vi "Assignment.vi"() -> ()   [LabVIEW 2023]
uses:
  Control 1.ctl
  Control 2.ctl
panel:
  in  "Tab Control":enum32{"Page 1", "Page 2", "Page 3"}(tab)
  out "seconds":string
  out "welcome":string
  out "Move Back":bool
  out "Move Forward":bool
  out "Vehicle Out of Position":bool
  out "Air Dry":bool
  out "Clear Water Rinse":bool
  out "Main High Pressure Wash":bool
  out "Soap Application":bool
  out "Under Body Wash":bool
  in  "Air Dry\nPosition \nSwitch":bool
  in  "Main Wash\nPosition\nSwitch":bool
  in  "Under Body\nWash Position\nSwitch":bool
  in  "Economy Wash":bool
  in  "Deluxe Wash":bool
  in  "stop":bool
  out "Next cycle in:":dbl format="%#.2f"
  out "Current Cycle:":string
  in  "Guest":bool
  in  "Login":bool
  in  "Password:":string
  in  "Username:":string
  # "Car Wash indicators"
  # "Car Wash Simulation Switches"
  # "Purchase Selection"
  # "Welcome to Touchless Carwash"
  # "Wash Complete! Drive Safely."
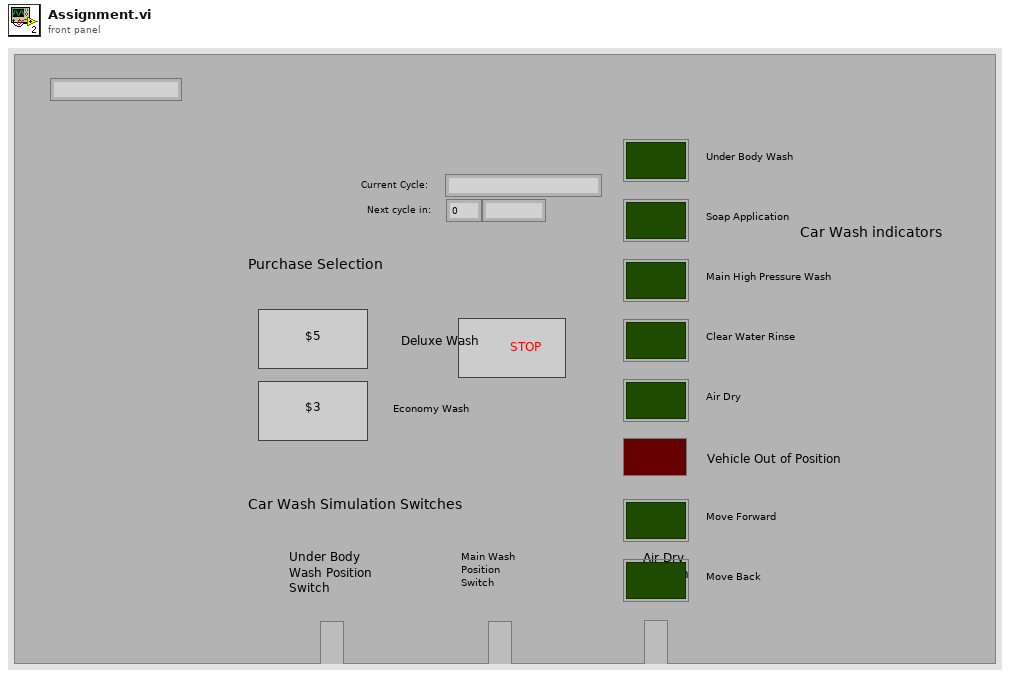
[diagram p1: front panel]
types:
  T1 = typedef "Control 1.ctl" = enum16{"init", "Login", "monitor switch", "monitor purchase selection", "decrement timer cycle", "Update cycle", "Logging"}
  T2 = enum8{"Enabled", "Disabled", "Disabled and Grayed Out"}
  T3 = typedef "Control 2.ctl" = enum16{"Under Body Wash", "Soap Application", "Main High Pressure Wash", "Clear Water Rinse", "Air Dry"}
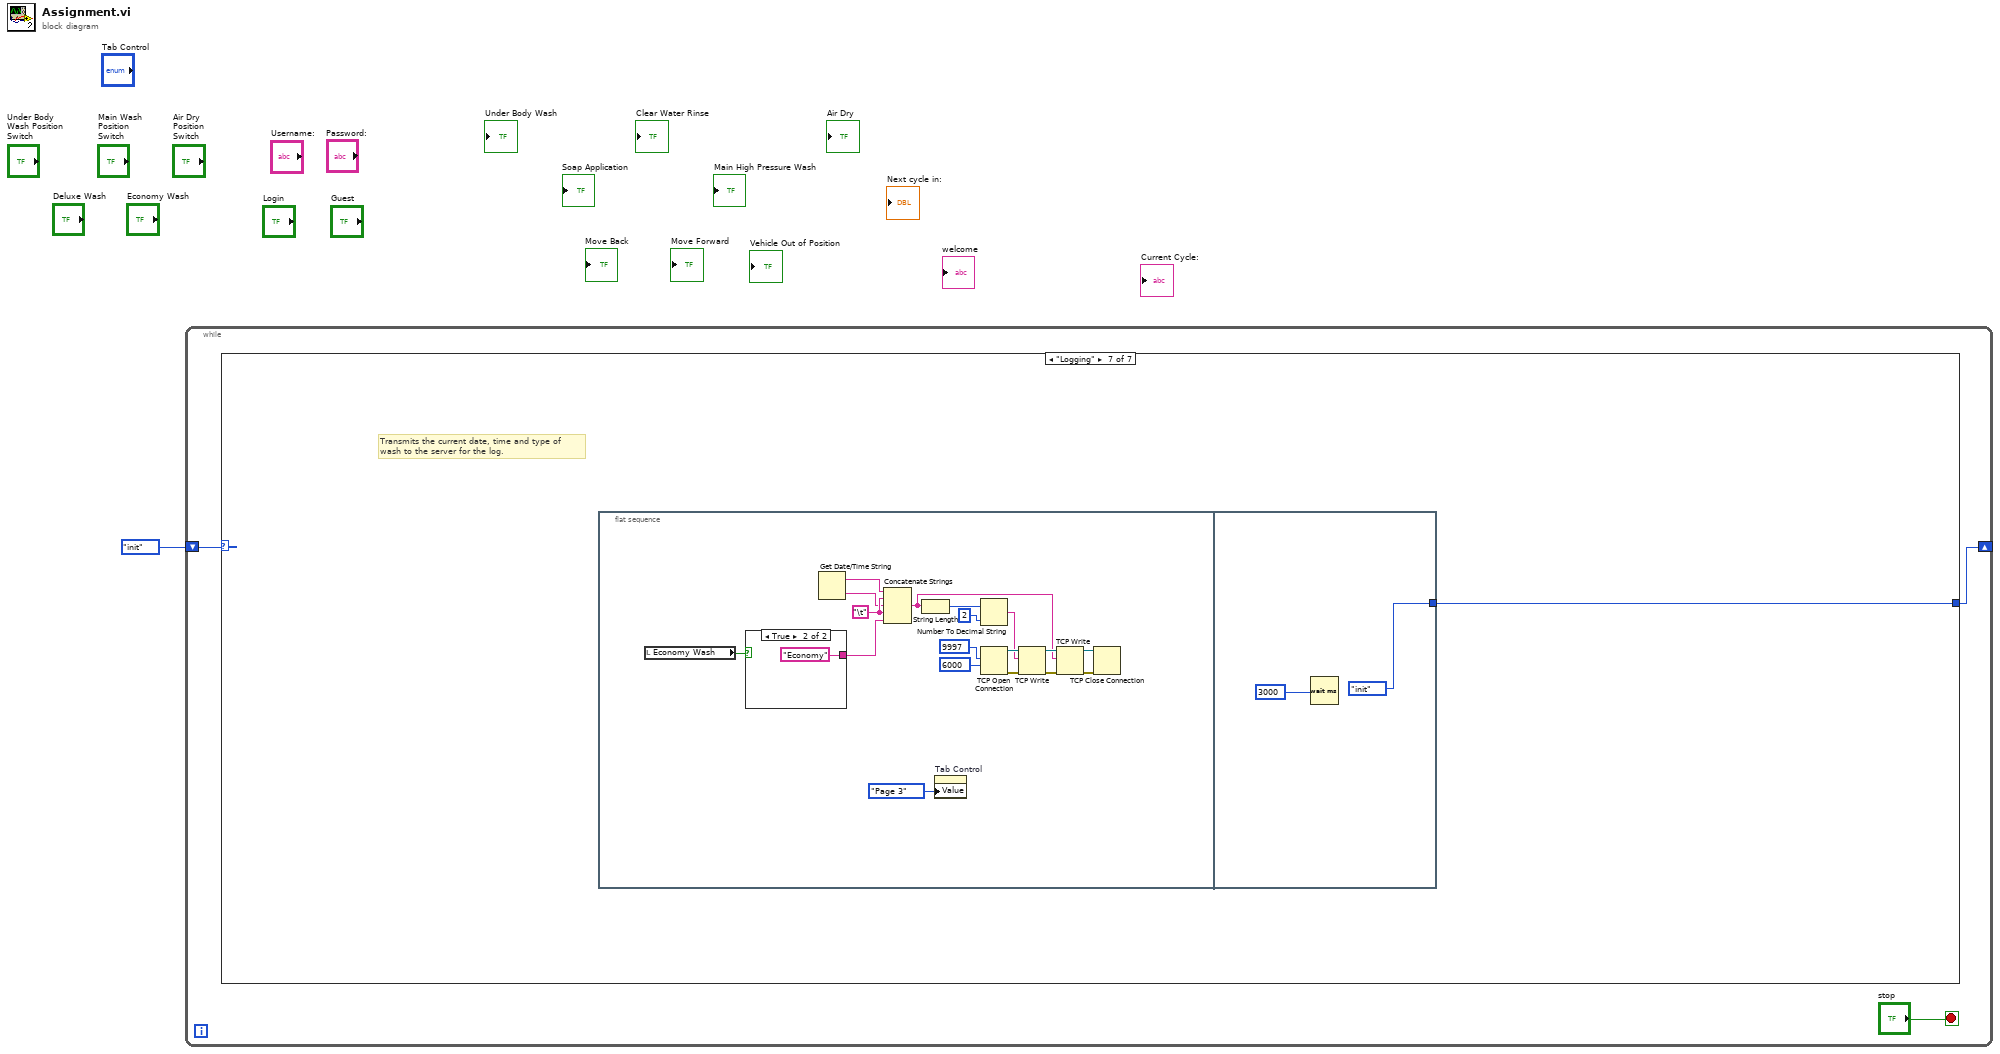
[diagram p0: block diagram]
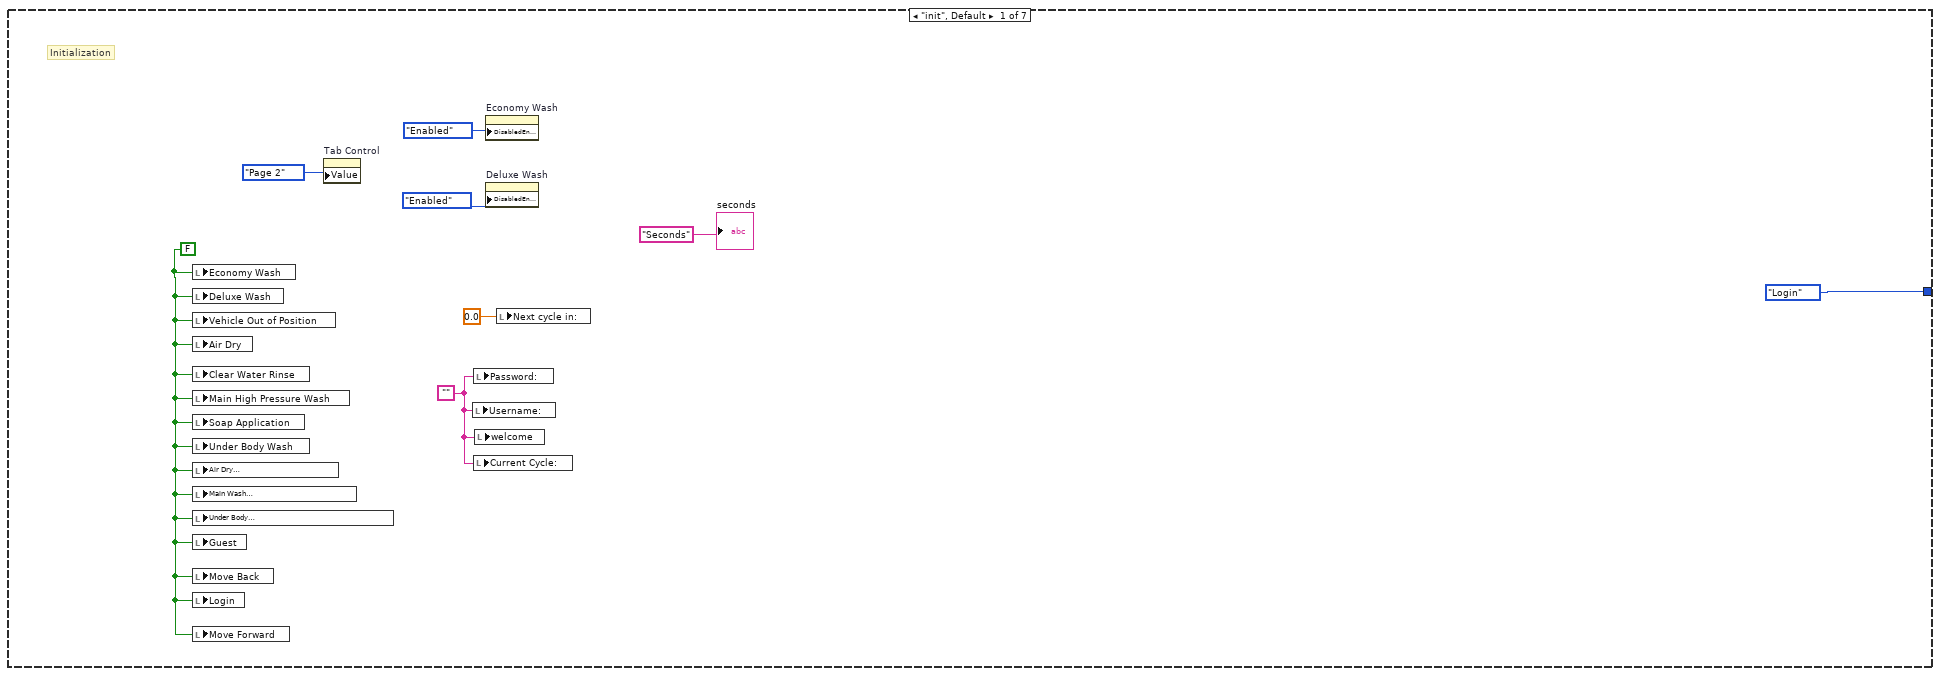
[diagram p2: hidden frame]
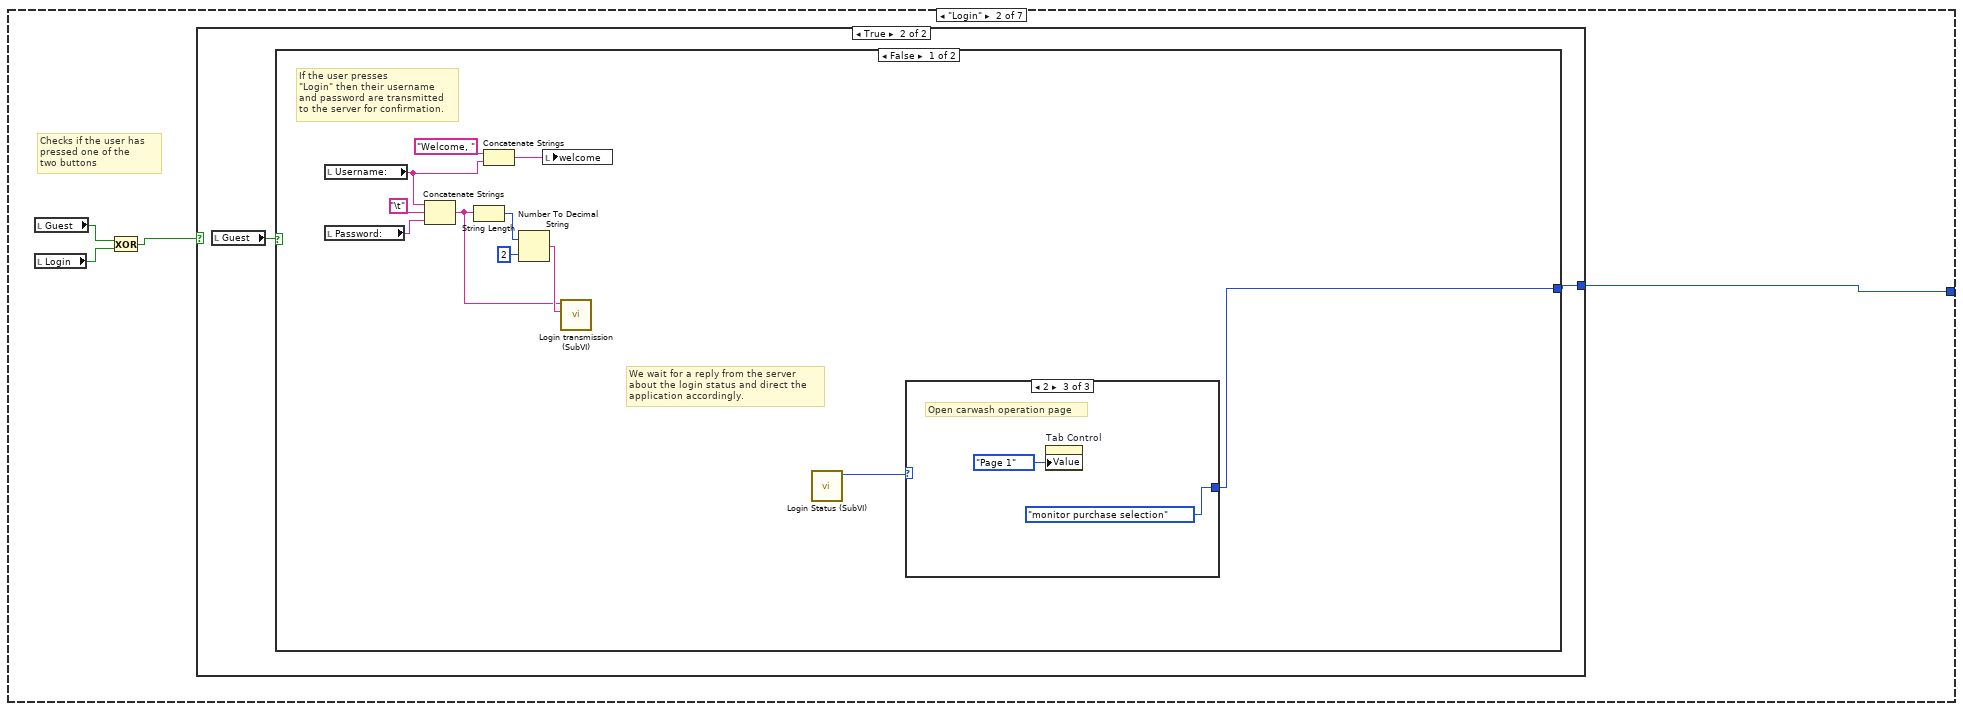
[diagram p3: hidden frame]
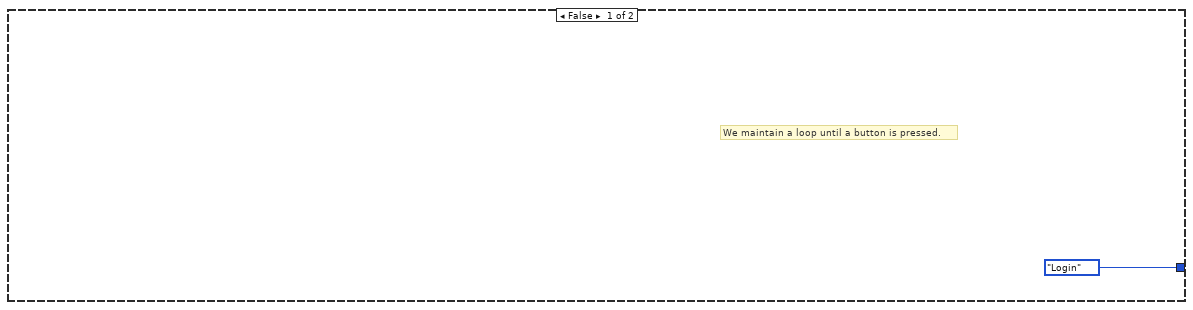
[diagram p4: hidden frame]
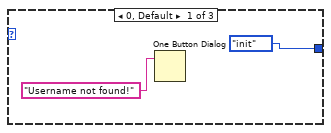
[diagram p5: hidden frame]
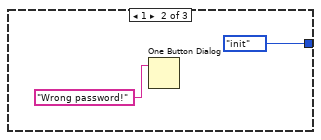
[diagram p6: hidden frame]
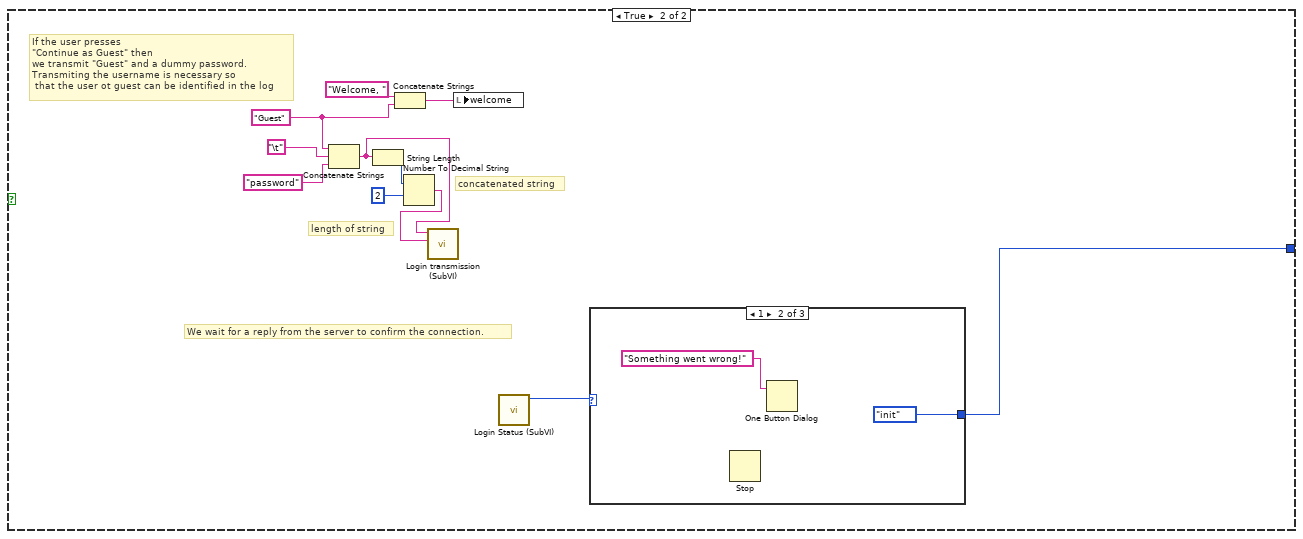
[diagram p7: hidden frame]
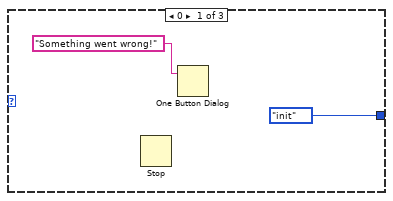
[diagram p8: hidden frame]
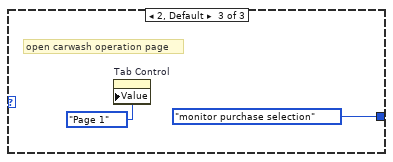
[diagram p9: hidden frame]
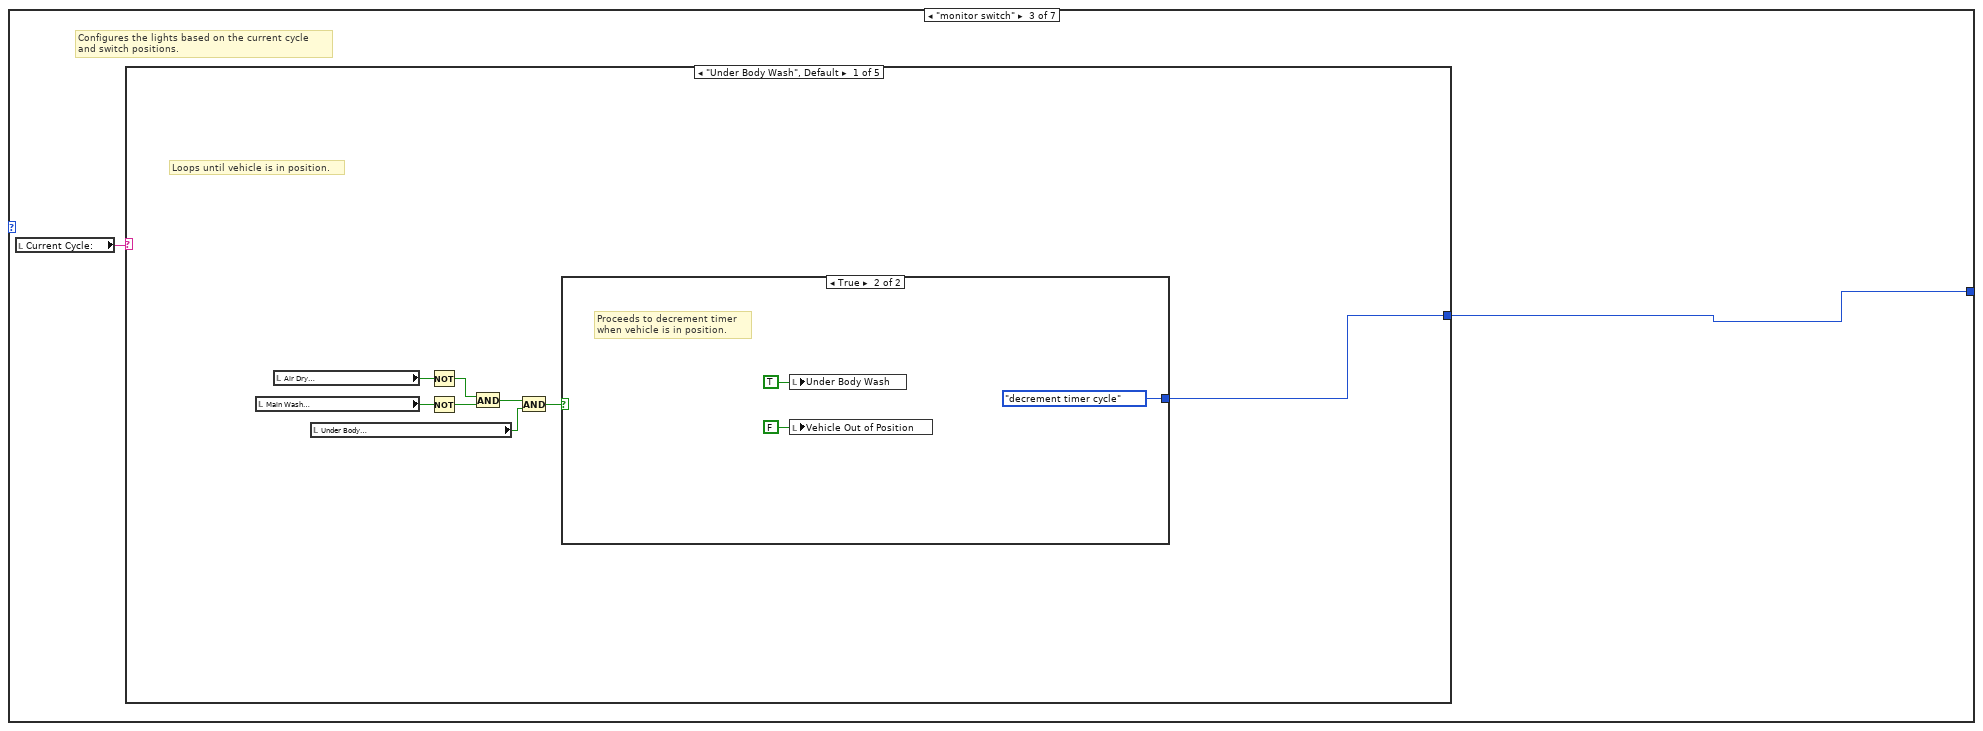
[diagram p10: hidden frame]
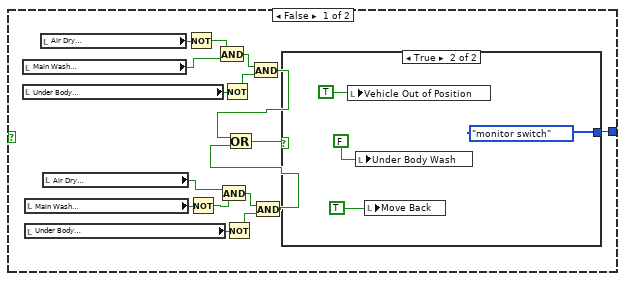
[diagram p11: hidden frame]
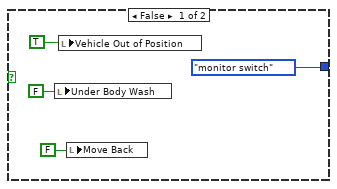
[diagram p12: hidden frame]
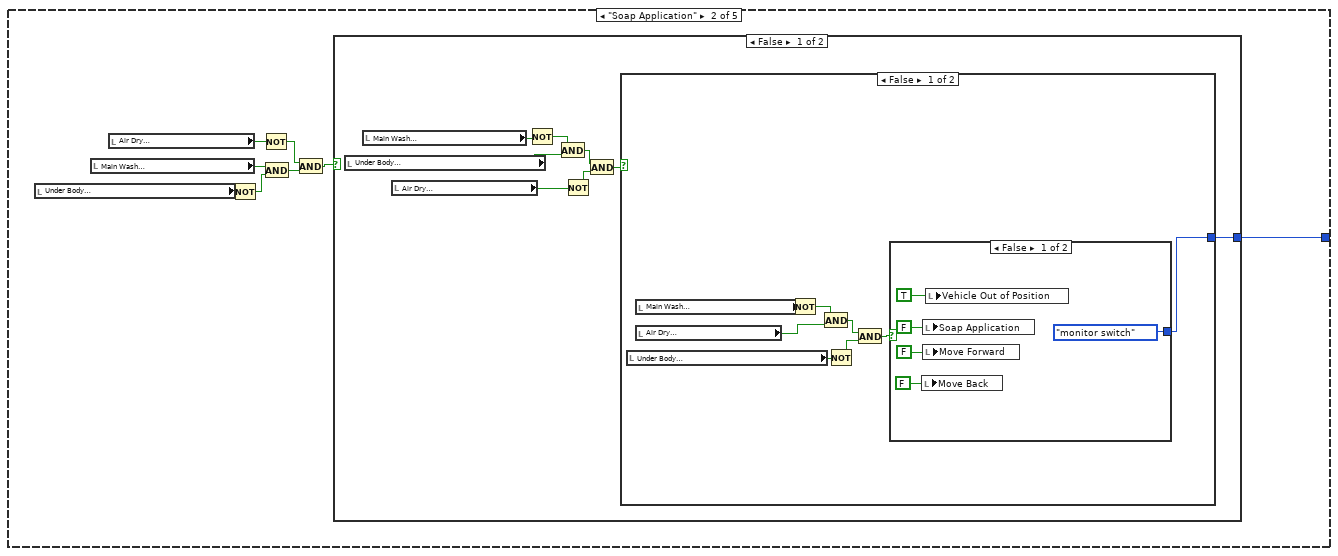
[diagram p13: hidden frame]
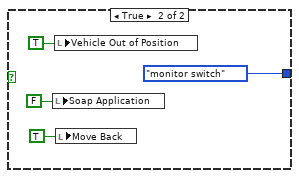
[diagram p14: hidden frame]
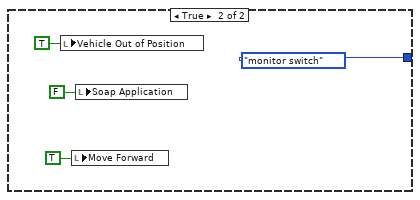
[diagram p15: hidden frame]
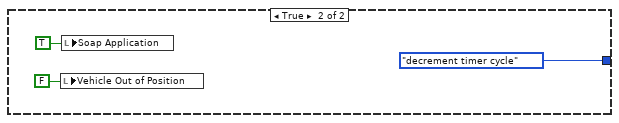
[diagram p16: hidden frame]
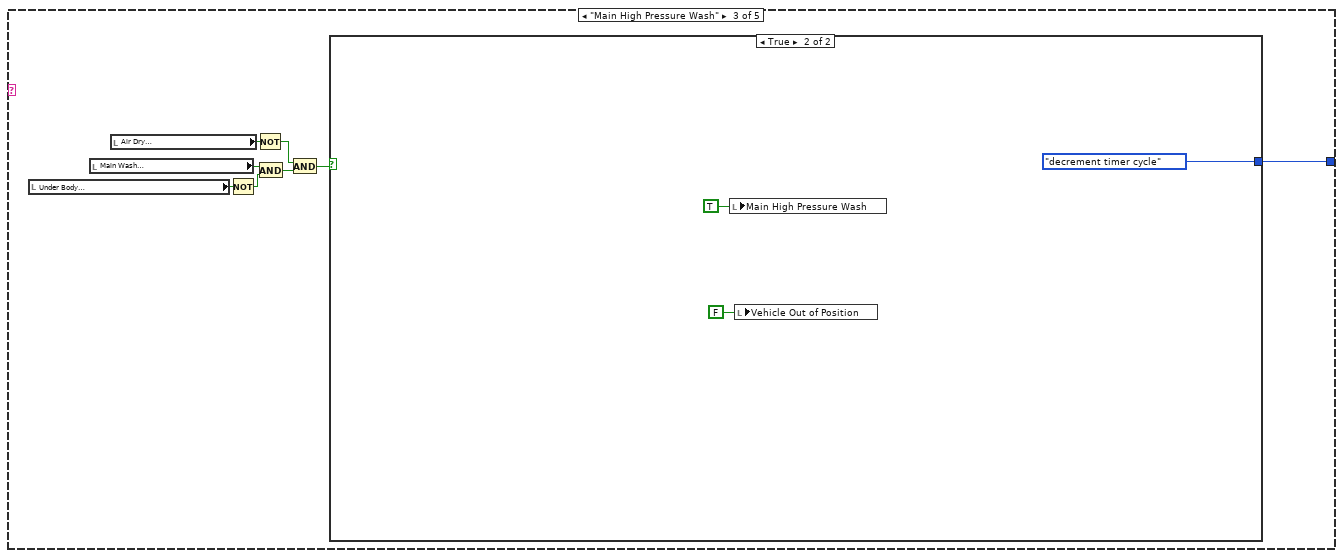
[diagram p17: hidden frame]
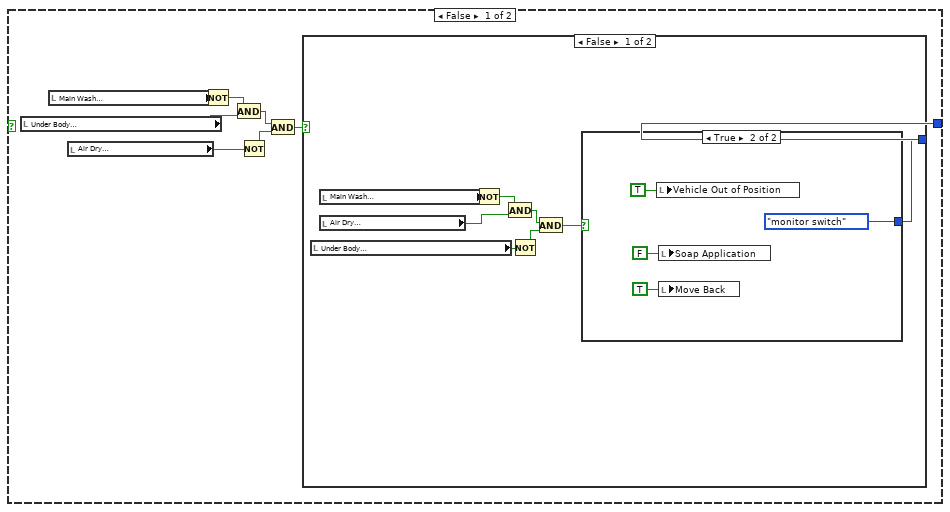
[diagram p18: hidden frame]
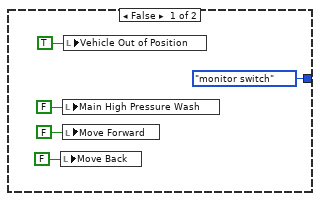
[diagram p19: hidden frame]
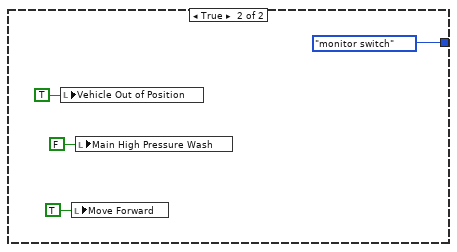
[diagram p20: hidden frame]
diagram:
  n1 = while {
    shift-right: [w3] -> _
    shift-left: Control_1."init" -> [w2]
    stop <- "stop" stop-if-true
    n2 = case shown="\"Logging\"" w2 {
      tunnel: [Control_1."Login" w13 w55 w246 Control_1."Update cycle" w270 w301] -> w3
      frame "init", Default {
        w5 = ""
        w7 = FALSE
        # "Initialization"
        n3 = local write "Economy Wash"(w7) -> ()
        n4 = local write "Deluxe Wash"(w7) -> ()
        n5 = local write "Vehicle Out of Position"(w7) -> ()
        n6 = local write "Air Dry"(w7) -> ()
        n7 = local write "Clear Water Rinse"(w7) -> ()
        n8 = local write "Main High Pressure Wash"(w7) -> ()
        n9 = local write "Soap Application"(w7) -> ()
        n10 = local write "Under Body Wash"(w7) -> ()
        n11 = local write "Air Dry\nPosition \nSwitch"(w7) -> ()
        n12 = local write "Main Wash\nPosition\nSwitch"(w7) -> ()
        n13 = local write "Under Body\nWash Position\nSwitch"(w7) -> ()
        n14 = local write "Guest"(w7) -> ()
        n15 = local write "Move Back"(w7) -> ()
        n16 = local write "Login"(w7) -> ()
        n17 = local write "Move Forward"(w7) -> ()
        n18 = property on="Tab Control" class="TabCtl (strict)"("Value"=enum32{"Page 1", "Page 2"}."Page 2" ("Tab Control")) -> ()  [unwired: 2 in, 2 out]
        n19 = local write "Username:"(w5) -> ()
        n20 = local write "Password:"(w5) -> ()
        n21 = local write "Current Cycle:"(w5) -> ()
        n22 = local write "welcome"(w5) -> ()
        n23 = property on="Economy Wash" class="Bool (strict)"("DisabledEnum"=T2."Enabled" ("Disabled")) -> ()  [unwired: 2 in, 2 out]
        n24 = property on="Deluxe Wash" class="Bool (strict)"("DisabledEnum"=T2."Enabled" ("Disabled")) -> ()  [unwired: 2 in, 2 out]
        n25 = local write "Next cycle in:"(0.0 ("Timer")) -> ()
        "seconds" <- "Seconds" ("seconds")
      }
      frame "Login" {
        # "Checks if the user has \npressed one of the\ntwo buttons"
        n26 = local read "Guest"() -> (w15:bool)
        n27 = local read "Login"() -> (w14:bool)
        n28 = Exclusive Or(1:w14, 2:w15) -> (0:w16:bool)
        n29 = case shown="True" w16 {
          tunnel: [Control_1."Login" w18] -> w13
          frame False {
            # "We maintain a loop until a button is pressed."
          }
          frame True {
            n30 = local read "Guest"() -> (w19:bool)
            n31 = case shown="False" w19 {
              tunnel: [w26 w43] -> w18
              frame False {
                # "We wait for a reply from the server\nabout the login status and direct the \napplication accordingly."
                # "If the user presses \n\"Login\" then their username \nand password are transmitted\nto the server for confirmation."
                n32 = local read "Username:"() -> (w21:string)
                n33 = local read "Password:"() -> (w30:string)
                n34 = Concatenate Strings(w21, "\t", w30) -> (w24:string)
                n35 = String Length(string=w24) -> (length=w29:i32)
                n36 = Concatenate Strings("Welcome, " ("string"), w21) -> (w22:string)
                n37 = Number To Decimal String(number=w29, width (-)=i16 2) -> (decimal integer string=w28:string)
                n38 = local write "welcome"(w22) -> ()
                n39 = call "Login transmission (SubVI).vi"("length of string"=w28, "String"=w24) -> ()  [unwired: 10 in]
                n40 = call "Login Status (SubVI).vi"() -> ("Numeric"=w20:i32)  [unwired: 11 in]
                n41 = case shown="2" w20 {
                  tunnel: [Control_1."init" Control_1."init" Control_1."monitor purchase selection"] -> w26
                  frame 0, Default {
                    n42 = One Button Dialog(message="Username not found!") -> ()  [unwired: 1 in, 1 out]
                  }
                  frame 1 {
                    n43 = One Button Dialog(message="Wrong password!") -> ()  [unwired: 1 in, 1 out]
                  }
                  frame 2 {
                    # "Open carwash operation page"
                    n44 = property on="Tab Control" class="TabCtl (strict)"("Value"=enum32{"Page 1", "Page 2"}."Page 1" ("Tab Control")) -> ()  [unwired: 2 in, 2 out]
                  }
                }
              }
              frame True {
                w37 = "Guest" ("string")
                # "concatenated string"
                # "length of string"
                # "We wait for a reply from the server to confirm the connection."
                # "If the user presses \n\"Continue as Guest\" then\nwe transmit \"Guest\" and a dummy password.\nTransmiting the username is necessary so\n that the user ot guest can be identified in the log"
                n45 = Concatenate Strings(w37, "\t", "password" ("string")) -> (w40:string)
                n46 = String Length(string=w40) -> (length=w47:i32)
                n47 = Concatenate Strings("Welcome, " ("string"), w37) -> (w39:string)
                n48 = Number To Decimal String(number=w47, width (-)=i16 2) -> (decimal integer string=w41:string)
                n49 = call "Login transmission (SubVI).vi"("length of string"=w41, "String"=w40) -> ()  [unwired: 10 in]
                n50 = local write "welcome"(w39) -> ()
                n51 = call "Login Status (SubVI).vi"() -> ("Numeric"=w46:i32)  [unwired: 11 in]
                n52 = case shown="1" w46 {
                  tunnel: [Control_1."init" Control_1."init" Control_1."monitor purchase selection"] -> w43
                  frame 0 {
                    n53 = Stop() -> ()  [unwired: 1 in]
                    n54 = One Button Dialog(message="Something went wrong!") -> ()  [unwired: 1 in, 1 out]
                  }
                  frame 1 {
                    n55 = Stop() -> ()  [unwired: 1 in]
                    n56 = One Button Dialog(message="Something went wrong!") -> ()  [unwired: 1 in, 1 out]
                  }
                  frame 2, Default {
                    # "open carwash operation page"
                    n57 = property on="Tab Control" class="TabCtl (strict)"("Value"=enum32{"Page 1", "Page 2"}."Page 1" ("Tab Control")) -> ()  [unwired: 2 in, 2 out]
                  }
                }
              }
            }
          }
        }
      }
      frame "monitor switch" {
        # "Configures the lights based on the current cycle\nand switch positions."
        n58 = local read "Current Cycle:"() -> (w54:string)
        n59 = case shown="\"Under Body Wash\", Default" w54 {
          tunnel: [w56 w92 w132 w172 w211] -> w55
          frame "Under Body Wash", Default {
            # "Loops until vehicle is in position."
            n60 = local read "Main Wash\nPosition\nSwitch"() -> (w63:bool)
            n61 = local read "Air Dry\nPosition \nSwitch"() -> (w62:bool)
            n62 = local read "Under Body\nWash Position\nSwitch"() -> (w59:bool)
            n63 = Not(x=w62) -> (.not. x?=w61:bool)
            n64 = Not(x=w63) -> (.not. x?=w60:bool)
            n65 = And(x=w61, y=w60) -> (x .and. y?=w58:bool)
            n66 = And(x=w58, y=w59) -> (x .and. y?=w57:bool)
            n67 = case shown="True" w57 {
              tunnel: [w65 Control_1."decrement timer cycle"] -> w56
              frame False {
                n68 = local read "Main Wash\nPosition\nSwitch"() -> (w76:bool)
                n69 = local read "Under Body\nWash Position\nSwitch"() -> (w79:bool)
                n70 = local read "Main Wash\nPosition\nSwitch"() -> (w70:bool)
                n71 = local read "Under Body\nWash Position\nSwitch"() -> (w71:bool)
                n72 = local read "Air Dry\nPosition \nSwitch"() -> (w78:bool)
                n73 = local read "Air Dry\nPosition \nSwitch"() -> (w69:bool)
                n74 = Not(x=w78) -> (.not. x?=w77:bool)
                n75 = Not(x=w70) -> (.not. x?=w68:bool)
                n76 = And(x=w77, y=w76) -> (x .and. y?=w74:bool)
                n77 = And(x=w69, y=w68) -> (x .and. y?=w73:bool)
                n78 = Not(x=w79) -> (.not. x?=w75:bool)
                n79 = Not(x=w71) -> (.not. x?=w72:bool)
                n80 = And(x=w74, y=w75) -> (x .and. y?=w67:bool)
                n81 = And(x=w73, y=w72) -> (x .and. y?=w66:bool)
                n82 = Or(x=w67, y=w66) -> (x .or. y?=w64:bool)
                n83 = case shown="True" w64 {
                  tunnel: [Control_1."monitor switch" Control_1."monitor switch"] -> w65
                  frame False {
                    n84 = local write "Under Body Wash"(FALSE ("Under Body Wash")) -> ()
                    n85 = local write "Vehicle Out of Position"(TRUE ("Vehicle Out of Position")) -> ()
                    n86 = local write "Move Back"(FALSE ("Move Back")) -> ()
                  }
                  frame True {
                    n87 = local write "Vehicle Out of Position"(TRUE ("Vehicle Out of Position")) -> ()
                    n88 = local write "Under Body Wash"(FALSE ("Under Body Wash")) -> ()
                    n89 = local write "Move Back"(TRUE ("Move Back")) -> ()
                  }
                }
              }
              frame True {
                # "Proceeds to decrement timer\nwhen vehicle is in position."
                n90 = local write "Under Body Wash"(TRUE ("Under Body Wash")) -> ()
                n91 = local write "Vehicle Out of Position"(FALSE ("Vehicle Out of Position")) -> ()
              }
            }
          }
          frame "Soap Application" {
            n92 = local read "Under Body\nWash Position\nSwitch"() -> (w98:bool)
            n93 = local read "Main Wash\nPosition\nSwitch"() -> (w95:bool)
            n94 = local read "Air Dry\nPosition \nSwitch"() -> (w97:bool)
            n95 = Not(x=w98) -> (.not. x?=w96:bool)
            n96 = Not(x=w97) -> (.not. x?=w93:bool)
            n97 = And(x=w95, y=w96) -> (x .and. y?=w94:bool)
            n98 = And(x=w93, y=w94) -> (x .and. y?=w91:bool)
            n99 = case shown="False" w91 {
              tunnel: [w99 Control_1."decrement timer cycle"] -> w92
              frame False {
                n100 = local read "Under Body\nWash Position\nSwitch"() -> (w103:bool)
                n101 = local read "Main Wash\nPosition\nSwitch"() -> (w105:bool)
                n102 = local read "Air Dry\nPosition \nSwitch"() -> (w106:bool)
                n103 = Not(x=w105) -> (.not. x?=w104:bool)
                n104 = And(x=w104, y=w103) -> (x .and. y?=w101:bool)
                n105 = Not(x=w106) -> (.not. x?=w102:bool)
                n106 = And(x=w101, y=w102) -> (x .and. y?=w100:bool)
                n107 = case shown="False" w100 {
                  tunnel: [w108 Control_1."monitor switch"] -> w99
                  frame False {
                    n108 = local read "Under Body\nWash Position\nSwitch"() -> (w109:bool)
                    n109 = local read "Main Wash\nPosition\nSwitch"() -> (w110:bool)
                    n110 = local read "Air Dry\nPosition \nSwitch"() -> (w112:bool)
                    n111 = Not(x=w110) -> (.not. x?=w111:bool)
                    n112 = And(x=w111, y=w112) -> (x .and. y?=w114:bool)
                    n113 = Not(x=w109) -> (.not. x?=w113:bool)
                    n114 = And(x=w114, y=w113) -> (x .and. y?=w107:bool)
                    n115 = case shown="False" w107 {
                      tunnel: [Control_1."monitor switch" Control_1."monitor switch"] -> w108
                      frame False {
                        n116 = local write "Move Back"(FALSE ("Move Back")) -> ()
                        n117 = local write "Soap Application"(FALSE ("Under Body Wash")) -> ()
                        n118 = local write "Move Forward"(FALSE ("Move Back")) -> ()
                        n119 = local write "Vehicle Out of Position"(TRUE ("Vehicle Out of Position")) -> ()
                      }
                      frame True {
                        n120 = local write "Soap Application"(FALSE ("Under Body Wash")) -> ()
                        n121 = local write "Vehicle Out of Position"(TRUE ("Vehicle Out of Position")) -> ()
                        n122 = local write "Move Back"(TRUE ("Move Back")) -> ()
                      }
                    }
                  }
                  frame True {
                    n123 = local write "Vehicle Out of Position"(TRUE ("Vehicle Out of Position")) -> ()
                    n124 = local write "Move Forward"(TRUE ("Move Back")) -> ()
                    n125 = local write "Soap Application"(FALSE ("Under Body Wash")) -> ()
                  }
                }
              }
              frame True {
                n126 = local write "Vehicle Out of Position"(FALSE ("Vehicle Out of Position")) -> ()
                n127 = local write "Soap Application"(TRUE ("Soap Application")) -> ()
              }
            }
          }
          frame "Main High Pressure Wash" {
            n128 = local read "Under Body\nWash Position\nSwitch"() -> (w138:bool)
            n129 = local read "Main Wash\nPosition\nSwitch"() -> (w135:bool)
            n130 = local read "Air Dry\nPosition \nSwitch"() -> (w137:bool)
            n131 = Not(x=w138) -> (.not. x?=w136:bool)
            n132 = Not(x=w137) -> (.not. x?=w133:bool)
            n133 = And(x=w135, y=w136) -> (x .and. y?=w134:bool)
            n134 = And(x=w133, y=w134) -> (x .and. y?=w131:bool)
            n135 = case shown="True" w131 {
              tunnel: [w139 Control_1."decrement timer cycle"] -> w132
              frame False {
                n136 = local read "Under Body\nWash Position\nSwitch"() -> (w143:bool)
                n137 = local read "Main Wash\nPosition\nSwitch"() -> (w145:bool)
                n138 = local read "Air Dry\nPosition \nSwitch"() -> (w146:bool)
                n139 = Not(x=w145) -> (.not. x?=w144:bool)
                n140 = And(x=w144, y=w143) -> (x .and. y?=w141:bool)
                n141 = Not(x=w146) -> (.not. x?=w142:bool)
                n142 = And(x=w141, y=w142) -> (x .and. y?=w140:bool)
                n143 = case shown="False" w140 {
                  tunnel: [w148 Control_1."monitor switch"] -> w139
                  frame False {
                    n144 = local read "Under Body\nWash Position\nSwitch"() -> (w149:bool)
                    n145 = local read "Main Wash\nPosition\nSwitch"() -> (w150:bool)
                    n146 = local read "Air Dry\nPosition \nSwitch"() -> (w152:bool)
                    n147 = Not(x=w150) -> (.not. x?=w151:bool)
                    n148 = And(x=w151, y=w152) -> (x .and. y?=w154:bool)
                    n149 = Not(x=w149) -> (.not. x?=w153:bool)
                    n150 = And(x=w154, y=w153) -> (x .and. y?=w147:bool)
                    n151 = case shown="True" w147 {
                      tunnel: [Control_1."monitor switch" Control_1."monitor switch"] -> w148
                      frame False {
                        n152 = local write "Move Back"(FALSE ("Move Back")) -> ()
                        n153 = local write "Main High Pressure Wash"(FALSE ("Under Body Wash")) -> ()
                        n154 = local write "Move Forward"(FALSE ("Move Back")) -> ()
                        n155 = local write "Vehicle Out of Position"(TRUE ("Vehicle Out of Position")) -> ()
                      }
                      frame True {
                        n156 = local write "Vehicle Out of Position"(TRUE ("Vehicle Out of Position")) -> ()
                        n157 = local write "Soap Application"(FALSE ("Under Body Wash")) -> ()
                        n158 = local write "Move Back"(TRUE ("Move Back")) -> ()
                      }
                    }
                  }
                  frame True {
                    n159 = local write "Vehicle Out of Position"(TRUE ("Vehicle Out of Position")) -> ()
                    n160 = local write "Move Forward"(TRUE ("Move Back")) -> ()
                    n161 = local write "Main High Pressure Wash"(FALSE ("Under Body Wash")) -> ()
                  }
                }
              }
              frame True {
                n162 = local write "Main High Pressure Wash"(TRUE ("Soap Application")) -> ()
                n163 = local write "Vehicle Out of Position"(FALSE ("Vehicle Out of Position")) -> ()
              }
            }
          }
          frame "Clear Water Rinse" {
            n164 = local read "Under Body\nWash Position\nSwitch"() -> (w178:bool)
            n165 = local read "Main Wash\nPosition\nSwitch"() -> (w175:bool)
            n166 = local read "Air Dry\nPosition \nSwitch"() -> (w177:bool)
            n167 = Not(x=w178) -> (.not. x?=w176:bool)
            n168 = Not(x=w177) -> (.not. x?=w173:bool)
            n169 = And(x=w175, y=w176) -> (x .and. y?=w174:bool)
            n170 = And(x=w173, y=w174) -> (x .and. y?=w171:bool)
            n171 = case shown="False" w171 {
              tunnel: [w179 Control_1."decrement timer cycle"] -> w172
              frame False {
                n172 = local read "Under Body\nWash Position\nSwitch"() -> (w183:bool)
                n173 = local read "Main Wash\nPosition\nSwitch"() -> (w185:bool)
                n174 = local read "Air Dry\nPosition \nSwitch"() -> (w186:bool)
                n175 = Not(x=w185) -> (.not. x?=w184:bool)
                n176 = And(x=w184, y=w183) -> (x .and. y?=w181:bool)
                n177 = Not(x=w186) -> (.not. x?=w182:bool)
                n178 = And(x=w181, y=w182) -> (x .and. y?=w180:bool)
                n179 = case shown="True" w180 {
                  tunnel: [w187 Control_1."monitor switch"] -> w179
                  frame False {
                    n180 = local read "Under Body\nWash Position\nSwitch"() -> (w189:bool)
                    n181 = local read "Main Wash\nPosition\nSwitch"() -> (w190:bool)
                    n182 = local read "Air Dry\nPosition \nSwitch"() -> (w192:bool)
                    n183 = Not(x=w190) -> (.not. x?=w191:bool)
                    n184 = And(x=w191, y=w192) -> (x .and. y?=w194:bool)
                    n185 = Not(x=w189) -> (.not. x?=w193:bool)
                    n186 = And(x=w194, y=w193) -> (x .and. y?=w188:bool)
                    n187 = case shown="False" w188 {
                      tunnel: [Control_1."monitor switch" Control_1."monitor switch"] -> w187
                      frame False {
                        n188 = local write "Vehicle Out of Position"(TRUE ("Vehicle Out of Position")) -> ()
                        n189 = local write "Clear Water Rinse"(FALSE ("Under Body Wash")) -> ()
                        n190 = local write "Move Forward"(FALSE ("Move Back")) -> ()
                        n191 = local write "Move Back"(FALSE ("Move Back")) -> ()
                      }
                      frame True {
                        n192 = local write "Clear Water Rinse"(FALSE ("Under Body Wash")) -> ()
                        n193 = local write "Vehicle Out of Position"(TRUE ("Vehicle Out of Position")) -> ()
                        n194 = local write "Move Back"(TRUE ("Move Back")) -> ()
                      }
                    }
                  }
                  frame True {
                    n195 = local write "Vehicle Out of Position"(TRUE ("Vehicle Out of Position")) -> ()
                    n196 = local write "Move Forward"(TRUE ("Move Back")) -> ()
                    n197 = local write "Clear Water Rinse"(FALSE ("Under Body Wash")) -> ()
                  }
                }
              }
              frame True {
                n198 = local write "Clear Water Rinse"(TRUE ("Soap Application")) -> ()
                n199 = local write "Vehicle Out of Position"(FALSE ("Vehicle Out of Position")) -> ()
              }
            }
          }
          frame "Air Dry" {
            n200 = local read "Under Body\nWash Position\nSwitch"() -> (w217:bool)
            n201 = local read "Main Wash\nPosition\nSwitch"() -> (w218:bool)
            n202 = local read "Air Dry\nPosition \nSwitch"() -> (w215:bool)
            n203 = Not(x=w218) -> (.not. x?=w216:bool)
            n204 = And(x=w215, y=w216) -> (x .and. y?=w214:bool)
            n205 = Not(x=w217) -> (.not. x?=w213:bool)
            n206 = And(x=w214, y=w213) -> (x .and. y?=w212:bool)
            n207 = case shown="False" w212 {
              tunnel: [w220 Control_1."decrement timer cycle"] -> w211
              frame False {
                n208 = local read "Under Body\nWash Position\nSwitch"() -> (w224:bool)
                n209 = local read "Main Wash\nPosition\nSwitch"() -> (w231:bool)
                n210 = local read "Under Body\nWash Position\nSwitch"() -> (w234:bool)
                n211 = local read "Main Wash\nPosition\nSwitch"() -> (w225:bool)
                n212 = local read "Air Dry\nPosition \nSwitch"() -> (w233:bool)
                n213 = local read "Air Dry\nPosition \nSwitch"() -> (w226:bool)
                n214 = Not(x=w233) -> (.not. x?=w232:bool)
                n215 = Not(x=w225) -> (.not. x?=w223:bool)
                n216 = And(x=w232, y=w231) -> (x .and. y?=w229:bool)
                n217 = And(x=w224, y=w223) -> (x .and. y?=w228:bool)
                n218 = Not(x=w234) -> (.not. x?=w230:bool)
                n219 = Not(x=w226) -> (.not. x?=w227:bool)
                n220 = And(x=w228, y=w227) -> (x .and. y?=w219:bool)
                n221 = And(x=w229, y=w230) -> (x .and. y?=w222:bool)
                n222 = Or(x=w222, y=w219) -> (x .or. y?=w221:bool)
                n223 = case shown="False" w221 {
                  tunnel: [Control_1."monitor switch" Control_1."monitor switch"] -> w220
                  frame False {
                    n224 = local write "Vehicle Out of Position"(TRUE ("Vehicle Out of Position")) -> ()
                    n225 = local write "Move Forward"(FALSE ("Move Back")) -> ()
                    n226 = local write "Air Dry"(FALSE ("Under Body Wash")) -> ()
                  }
                  frame True {
                    n227 = local write "Vehicle Out of Position"(TRUE ("Vehicle Out of Position")) -> ()
                    n228 = local write "Move Forward"(TRUE ("Move Back")) -> ()
                    n229 = local write "Air Dry"(FALSE ("Under Body Wash")) -> ()
                  }
                }
              }
              frame True {
                n230 = local write "Air Dry"(TRUE ("Soap Application")) -> ()
                n231 = local write "Vehicle Out of Position"(FALSE ("Vehicle Out of Position")) -> ()
              }
            }
          }
        }
      }
      frame "monitor purchase selection" {
        # "Checks if the user has pressed\none of the two buttons."
        n232 = local read "Economy Wash"() -> (w249:bool)
        n233 = local read "Deluxe Wash"() -> (w248:bool)
        n234 = Exclusive Or(1:w248, 2:w249) -> (0:w247:bool)
        n235 = case shown="True" w247 {
          tunnel: [Control_1."monitor purchase selection" w251] -> w246
          frame False {
            # "If no button is pressed then\nwe loop until a button is \npressed."
          }
          frame True {
            # "Disables both the buttons,\nand sets the intial cycle\nand timer based on the\nselection."
            n236 = local read "Deluxe Wash"() -> (w252:bool)
            n237 = case shown="False" w252 {
              tunnel: [Control_1."monitor switch" Control_1."monitor switch"] -> w251
              frame False {
                n238 = local write "Next cycle in:"(5.0 ("Timer")) -> ()
                n239 = property on="Deluxe Wash" class="Bool (strict)"("DisabledEnum"=T2."Disabled" ("Disabled")) -> ()  [unwired: 2 in, 2 out]
                n240 = property on="Economy Wash" class="Bool (strict)"("DisabledEnum"=T2."Disabled" ("Disabled")) -> ()  [unwired: 2 in, 2 out]
                n241 = Format Into String(Control_2."Soap Application") -> (resulting string=w253:string)  [unwired: 3 in, 1 out]
                n242 = local write "Current Cycle:"(w253) -> ()
              }
              frame True {
                n243 = local write "Next cycle in:"(10.0 ("Timer")) -> ()
                n244 = Format Into String(Control_2."Under Body Wash") -> (resulting string=w259:string)  [unwired: 3 in, 1 out]
                n245 = property on="Economy Wash" class="Bool (strict)"("DisabledEnum"=T2."Disabled" ("Disabled")) -> ()  [unwired: 2 in, 2 out]
                n246 = property on="Deluxe Wash" class="Bool (strict)"("DisabledEnum"=T2."Disabled" ("Disabled")) -> ()  [unwired: 2 in, 2 out]
                n247 = local write "Current Cycle:"(w259) -> ()
              }
            }
          }
        }
      }
      frame "decrement timer cycle" {
        # "The timer is decremented"
        n248 = local read "Next cycle in:"() -> (w268:dbl)
        n249 = Wait (ms)(milliseconds to wait=u32 5) -> ()  [unwired: 1 out]
        n250 = Subtract(x=w268, y=0.005) -> (x-y=w269:dbl)
        n251 = local write "Next cycle in:"(w269) -> ()
      }
      frame "Update cycle" {
        # "If the cycles have finished, then directs the\nprogram to logging."
        # "Updates the cycle if the timer has ran out."
        n252 = local read "Next cycle in:"() -> (w272:dbl)
        n253 = Less Or Equal To 0?(x=w272) -> (x <= 0?=w271:bool)
        n254 = case shown="True" w271 {
          tunnel: [Control_1."monitor switch" w275] -> w270
          frame False {
          }
          frame True {
            n255 = local read "Current Cycle:"() -> (w274:string)
            n256 = case shown="\"Air Dry\"" w274 {
              tunnel: [Control_1."monitor switch" Control_1."monitor switch" Control_1."monitor switch" w291 Control_1."Logging"] -> w275
              frame "Under Body Wash", Default {
                n257 = Format Into String(Control_2."Soap Application") -> (resulting string=w276:string)  [unwired: 3 in, 1 out]
                n258 = local write "Next cycle in:"(5.0 ("Timer")) -> ()
                n259 = local write "Under Body Wash"(FALSE ("Under Body Wash")) -> ()
                n260 = local write "Current Cycle:"(w276) -> ()
              }
              frame "Soap Application" {
                n261 = Format Into String(Control_2."Main High Pressure Wash") -> (resulting string=w281:string)  [unwired: 3 in, 1 out]
                n262 = local write "Next cycle in:"(5.0 ("Timer")) -> ()
                n263 = local write "Soap Application"(FALSE ("Under Body Wash")) -> ()
                n264 = local write "Current Cycle:"(w281) -> ()
              }
              frame "Main High Pressure Wash" {
                n265 = local write "Next cycle in:"(5.0 ("Timer")) -> ()
                n266 = local write "Main High Pressure Wash"(FALSE ("Under Body Wash")) -> ()
                n267 = Format Into String(Control_2."Clear Water Rinse") -> (resulting string=w287:string)  [unwired: 3 in, 1 out]
                n268 = local write "Current Cycle:"(w287) -> ()
              }
              frame "Clear Water Rinse" {
                n269 = local read "Economy Wash"() -> (w292:bool)
                n270 = case shown="False" w292 {
                  tunnel: [Control_1."monitor switch" Control_1."Logging"] -> w291
                  frame False {
                    n271 = local write "Clear Water Rinse"(FALSE ("Under Body Wash")) -> ()
                    n272 = local write "Next cycle in:"(10.0 ("Timer")) -> ()
                    n273 = Format Into String(Control_2."Air Dry") -> (resulting string=w293:string)  [unwired: 3 in, 1 out]
                    n274 = local write "Current Cycle:"(w293) -> ()
                  }
                  frame True {
                  }
                }
              }
              frame "Air Dry" {
                n275 = local write "Air Dry"(FALSE ("Air Dry")) -> ()
              }
            }
          }
        }
      }
      frame "Logging" {
        # "Transmits the current date, time and type of\nwash to the server for the log."
        n276 = flat-sequence {
          tunnel: [Control_1."init"] -> w301
          frame #0 {
            w307 = "\t"
            n277 = local read "Economy Wash"() -> (w312:bool)
            n278 = case shown="True" w312 {
              tunnel: ["Deluxe" "Economy"] -> w304
              frame False {
              }
              frame True {
              }
            }
            n279 = Get Date/Time String() -> (date string=w306:string, time string=w305:string)  [unwired: 3 in]
            n280 = Concatenate Strings(w306, w307, w305, w307, w304) -> (w308:string)
            n281 = String Length(string=w308) -> (length=w311:i32)
            n282 = property on="Tab Control" class="TabCtl (strict)"("Value"=enum32{"Page 1", "Page 2", "Page 3"}."Page 3" ("Tab Control")) -> ()  [unwired: 2 in, 2 out]
            n283 = Number To Decimal String(number=w311, width (-)=i16 2) -> (decimal integer string=w310:string)
            n284 = TCP Open Connection(remote port or service name=u16 9997, timeout ms (60000)=6000) -> (connection ID=w319:refnum<k5>, error out=w316:errorcluster)  [unwired: 3 in]
            n285 = TCP Write(connection ID=w319, data in=w310, error in (no error)=w316) -> (connection ID out=w318:refnum<k5>, error out=w315:errorcluster)  [unwired: 1 in, 1 out]
            n286 = TCP Write(connection ID=w318, data in=w308, error in (no error)=w315) -> (connection ID out=w317:refnum<k5>, error out=w314:errorcluster)  [unwired: 1 in, 1 out]
            n287 = TCP Close Connection(connection ID=w317, error in (no error)=w314) -> ()  [unwired: 1 in, 2 out]
          }
          frame #1 {
            n288 = Wait (ms)(milliseconds to wait=u32 3000) -> ()  [unwired: 1 out]
          }
        }
      }
    }
  }
